vi "global variable.vi"() -> ()   [LabVIEW 2017]
uses:
  <vilib>/addons/Sound and Vibration/Order Analysis/Ref Gabor Order Tracking/GT RefNum.ctl
  <vilib>/addons/Sound and Vibration/Order Analysis/Tach Process/SubVIs/speed profile.ctl
  <vilib>/addons/Sound and Vibration/Order Analysis/Gabor Order Tracking/SoundVib_Gabor.lvlib
  <vilib>/addons/Sound and Vibration/Order Analysis/Tach Process/SoundVib_TachProcess.lvlib
panel:
  out "pulses/rev":i32
  in  "EXE distribution?":bool
  out "Cfg File":path
  out "center freq":dbl[](array[numeric]) format="%.2f"
  out "Edge Information":T1 {"speed [RPM]" format="%.2f"; "time [s]" format="%.2f"}
  out "Gabor RefNum":T2
  out "sampling \nfrequency (Hz)":dbl
  out "window length":i32
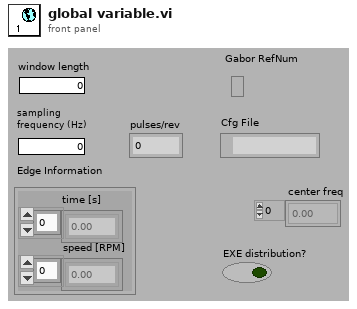
[diagram p1: front panel]
types:
  T1 = typedef "SoundVib_TachProcess.lvlib/speed profile.ctl" = cluster{"time [s]":dbl[], "speed [RPM]":dbl[]}
  T2 = typedef "SoundVib_Gabor.lvlib/GT RefNum.ctl" = refnum<k1>
diagram:
